vi "1_Dataset_Converter(Wave2STFT_PNG).vi"() -> ()   [LabVIEW 2020]
uses:
  Controls/Wave2STFT_Cfg.ctl
  <vilib>/Utility/libraryn.llb/Recursive File List.vi
  <vilib>/Utility/libraryn.llb/Get File Extension.vi
  subVIs/Read_Wav.vi
  subVIs/Spectrogram/Wf_to_STFT.vi
panel:
  out "error out":errorcluster
  out "Progress":i32
  out "Total":i32
  in  "Img. Res.":i32=128
  in  "STFT Config":T1={"FFT block size"=1024, "window"=3, "time segment"={"from [s]"=-1.0, "to [s]"=-1.0, "time increment"=20.0, "time increment units (%)"=enum."%"}, "dB On (T)"=TRUE, "Dynamic Range(dB)"=80.0, "Mel?"=TRUE} {"window" items=["None "=0, "Hanning"=1, "Hamming"=2, "Blackman-Harris"=3, "Exact Blackman"=4, "Blackman"=5, "Flat Top"=6, "4 Term B-Harris "=7, "7 Term B-Harris"=8, "Low Sidelobe"=9, "Blackman Nuttall"=11]}
  in  "Destination":path=path "D:/Data/DNN/Speech_Commands/data_speech_commands_v0.02_stft"
  in  "Source":path=path "D:/Data/DNN/Speech_Commands/data_speech_commands_v0.02"
  # "Overview: This code converts .wav files in the dataset into .png images of spectrograms.\nDataset: https://storage.cloud.google.com/download.tensorflow.org/data/speech_commands_v0.02.tar.gz\n\nRequirements:\n1. Deep Learning Toolkit for LabVIEW.\n2. NI Vision Development Module.\n3. Sound and Vibration Toolkit.\n\nInstructions:\n1. Download and extract the compressed wave dataset from the link above.\n2. Remove unnecessary files and folders, keeping only the folders containing the words (e.g., \"backward\", \"bed\", ... \"zero\") - a total of 35 folders/words.\n3. Provide the path to the wave dataset at \"Source\".\n4. Provide the path to the destination folder where the .png spectrograms will be stored.\n5. Run the VI. Note: This VI might take a couple of minutes to finish.\n6. Observe the generated spectrograms in the destination folder.\n7. Switch to the training VI in the project to proceed with training."
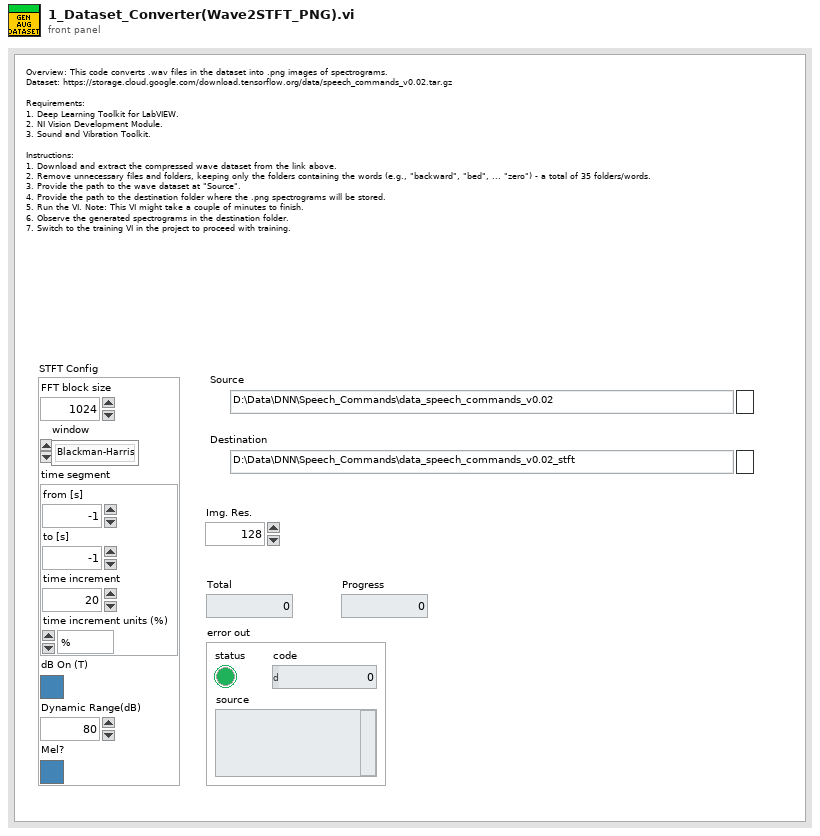
[diagram p1: front panel]
types:
  T1 = typedef "Wave2STFT_Cfg.ctl" = cluster{"FFT block size":i32, "window":u16, "time segment":cluster{"from [s]":dbl, "to [s]":dbl, "time increment":dbl, "time increment units (%)":enum16{"%", "s", "ms"}}, "dB On (T)":bool, "Dynamic Range(dB)":sgl, "Mel?":bool}
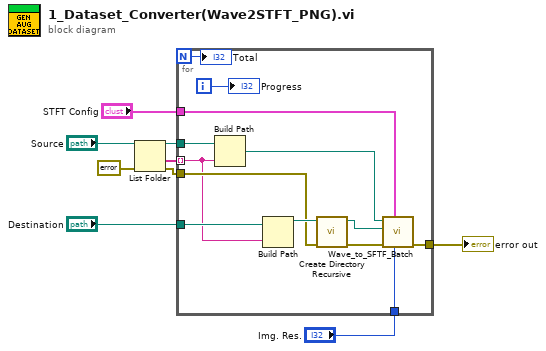
[diagram p0: block diagram]
diagram:
  n1 = List Folder(path="Source", error in=errorcluster {"status"=FALSE, "code"=0, "source"=""}) -> (path out=w6:path, folder names=w8:string[], error out=w4:errorcluster)  [unwired: 2 in, 1 out]
  n2 = for {
    N -> [w12]
    tunnel: "Destination" -> [w22]
    tunnel: [w21] -> w1
    tunnel: w6 -> [w20]
    tunnel: w8 -> [w13] mode=indexing
    tunnel: w4 -> [w17]
    tunnel: "STFT Config" -> [w15]
    tunnel: "Img. Res." -> [w14]
    i -> [w11]
    n3 = Build Path(base path=w20, name or relative path=w13) -> (appended path=w19:path)
    n4 = Build Path(base path=w22, name or relative path=w13) -> (appended path=w18:path)
    n5 = call <vilib>:"Create Directory Recursive.vi"("error in (no error)"=w17, "directory"=w18) -> ("error out"=w16:errorcluster, "directory copy"=w10:path)  [unwired: 3 in, 1 out]
    n6 = call "Wave_to_SFTF_Batch.vi"("Img. Res."=w14, "STFT Config"=w15, "error in (no error)"=w16, "path to dest."=w10, "path to wav"=w19) -> ("error out"=w21:errorcluster)  [unwired: 6 in]
    "Total" <- w12
    "Progress" <- w11
  }
  "error out" <- w1
